vi "bbauv_acoustic_sbRIO_v3.vi"() -> ()   [LabVIEW 2012]
doc: "This VI will initialize the FPGA VI and read a user-defined number of samples from a DMA FIFO. When the data acquisition is complete this VI will read status information from the FPGA VI.\n\nFollow these instructions to run the VI.\n\n1. Select your RIO device from the dropdown.\n2. Set the sample period, number of samples to acquire per channel, and DMA block read size. \n\nNote: the block read size should be set to balance load on the host processor and the update rate of the user interface. A small block read size will update the user interface more often but will result in a higher load on the host processor."
uses:
  <vilib>/userdefined/High Color/nirio_resource_hc.ctl
  <vilib>/Analysis/3filter.llb/Filter Passband Type.ctl
  <vilib>/FPGAPlugInAG/sbRIO-9612/niLvFpga_Open_sbRIO-9612.vi
  <vilib>/rvi/interface/common/dynamic/niFpgaDynamicAddResources.vi
  <vilib>/Utility/error.llb/Error Cluster From Error Code.vi
  <vilib>/FPGAPlugInAG/Dynamic/niLvFpga_Run_Dynamic.vi
  <vilib>/rvi/errors/niLvFpgaAdjustHostInterfaceError.vi
  <vilib>/RVI Host/nirviSupport.llb/nirviErrorClusterFromErrorCode.vi
  <vilib>/FPGAPlugInAG/Dynamic/niLvFpga_Close_Dynamic.vi
  <vilib>/Analysis/3filter.llb/Elliptic Filter (DBL).vi
  <vilib>/Analysis/3filter.llb/Butterworth Filter (DBL).vi
  <vilib>/rvi/interface/nirviOpenFPGA/nirviOpenFPGA.xnode
  FPGA Bitfiles/bbauvFPGA_FPGATarget2_NI9223User-Contr_AXBjtBmtN8Y.lvbitx
  NI 9223 User-Controlled IO Sampling (FPGA).vi
  <vilib>/rvi/interface/nirviMethod/nirviMethod.xnode
  <vilib>/rvi/interface/nirviReadWriteControl/nirviReadWriteControl.xnode
  <vilib>/rvi/interface/nirviCloseFPGA/nirviCloseFPGA.xnode
  <vilib>/rvi/errors/niLvFpgaMergeErrorWithErrorCode.vi
  <vilib>/rvi/interface/Simulation/niFpgaSimulationCallBeginRW.vi
  <vilib>/FPGAPlugInAG/Dynamic/niLvFpga_ReadFifo_Dynamic.vi
  <vilib>/rvi/interface/nirviMethod/StockFPGA_InlinedMethodWaitForSingleIRQ.vi
  <vilib>/FPGAPlugInAG/Dynamic/niLvFpga_WaitOnIrq_Dynamic.vi
  <vilib>/FPGAPlugInAG/Dynamic/niLvFpga_AcknowledgeIrq_Dynamic.vi
  NiFpgaLv.dll
  <vilib>/FPGAPlugInAG/Dynamic/niLvFpga_ConfigureFifo_Dynamic.vi
  <vilib>/FPGAPlugInAG/Dynamic/niLvFpga_StartFifo_Dynamic.vi
  <vilib>/Analysis/NI_AALBase.lvlib
panel:
  in  "Freq Lower Limit:":dbl=25000.0
  out "Selected Frequency:":dbl
  in  "Filter mode":enum16{"Elliptic", "Butterworth"}(ring)=enum."Butterworth"
  in  "Order":i32=3
  in  "Low Cutoff":dbl=20000.0
  in  "High Cutoff":dbl=26000.0
  in  "Freq Upper Limit:":dbl=25000.0
  out "Freq 2":dbl
  out "Freq 1":dbl
  in  "Noise length":i32=300
  out "Index 0":dbl
  out "Index 1":dbl
  out "Index 2":dbl
  out "Index 3":dbl
  out "amplitude 0":dbl
  out "amplitude 1":dbl
  out "amplitude 2":dbl
  out "amplitude 3":dbl
  in  "Portion Duration":i32=1000
  out "Threshold 0":dbl
  out "Threshold 1":dbl
  out "Threshold 2":dbl
  out "Threshold 3":dbl
  in  "threshold ratio":dbl=3.0
  in  "Display":bool
  in  "Sampling Duration (us)":u32=2005000
  in  "RIO Device":T1="RIO0"
  out "Timed Out":bool
  out "Sample Gated":bool
  out "Overwrite":bool
  in  "Acquisition Stop":bool
  out "Selected Index":i32
  out "Ratio at Index (%)":dbl
  in  "Threshold":dbl=0.3
  out "Original Filtered Ch0":dbl[](graph)
  out "bad signal?":bool
  out "dt1":dbl
  out "dt2":dbl
  out "dt3":dbl
  out "ROS  Error":bool
  in  "Send to ROS":bool=TRUE
  in  "Altitude":dbl=2.0
  out "x":dbl
  out "y":dbl
  out "z":dbl
  out "yaw":dbl
  out "pitch":dbl
  in  "Mode":T2(ring)=enum."Use Far Field"
  out "Forward":dbl
  out "Sidemove":dbl
  out "Arrival Analysis Signal":dbl[][](graph)
  out "Yaw Chart":dbl(graph)
  out "noise index":dbl[](array[numeric])
  out "Frequency Selected Signal":dbl[](graph)
  out "#Elements Acquired":u32(graph)
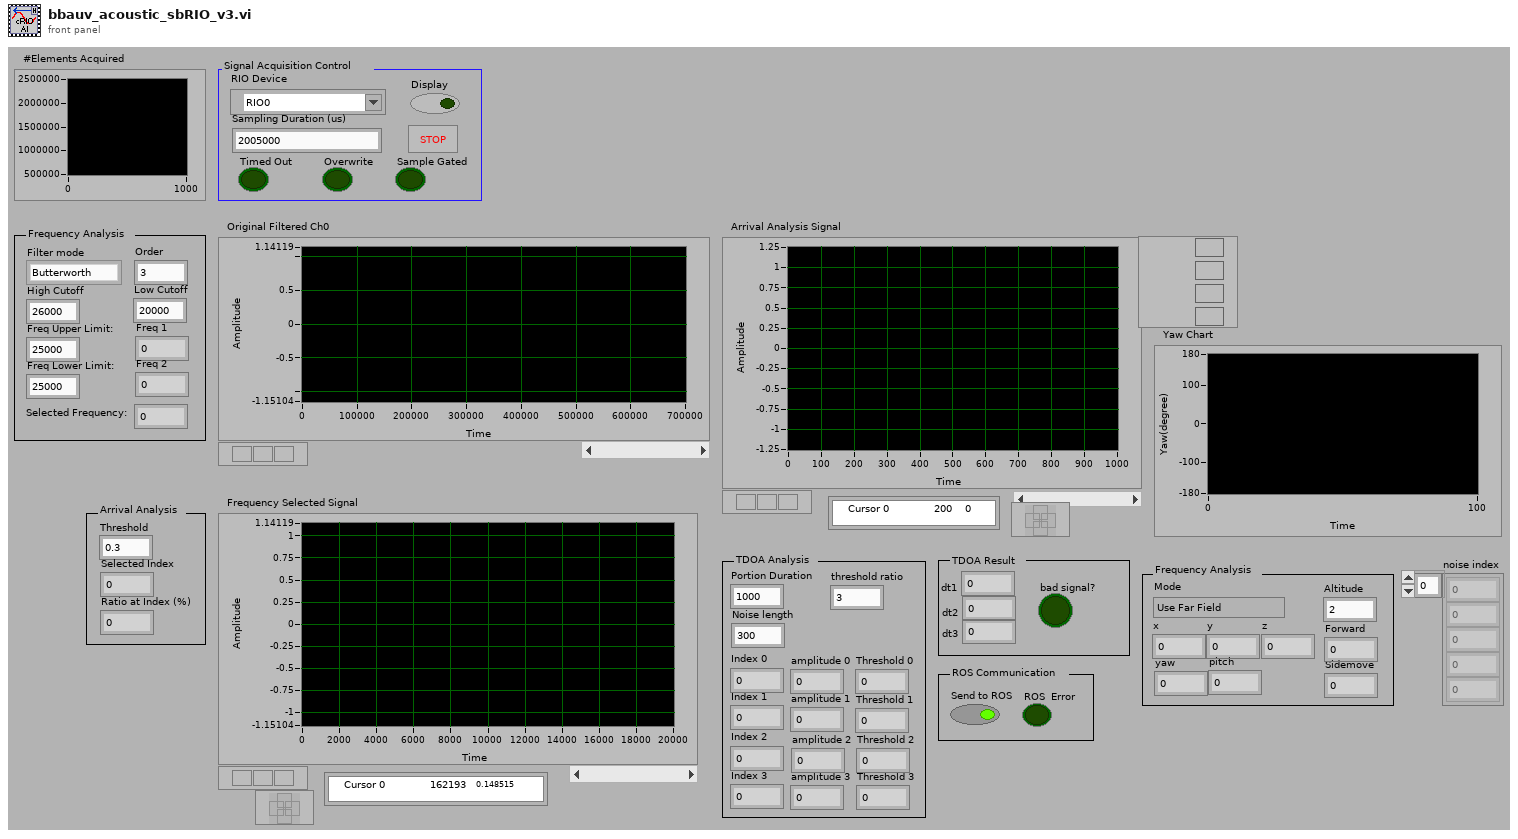
[diagram p1: front panel]
types:
  T1 = typedef "nirio_resource_hc.ctl" = tag
  T2 = enum16{"Use Near Field", "Use Far Field", "Far Field with 3 hydrophones"}
  T3 = typedef "NI_AALBase.lvlib/Filter Passband Type.ctl" = enum32{"Lowpass", "Highpass", "Bandpass", "Bandstop"}
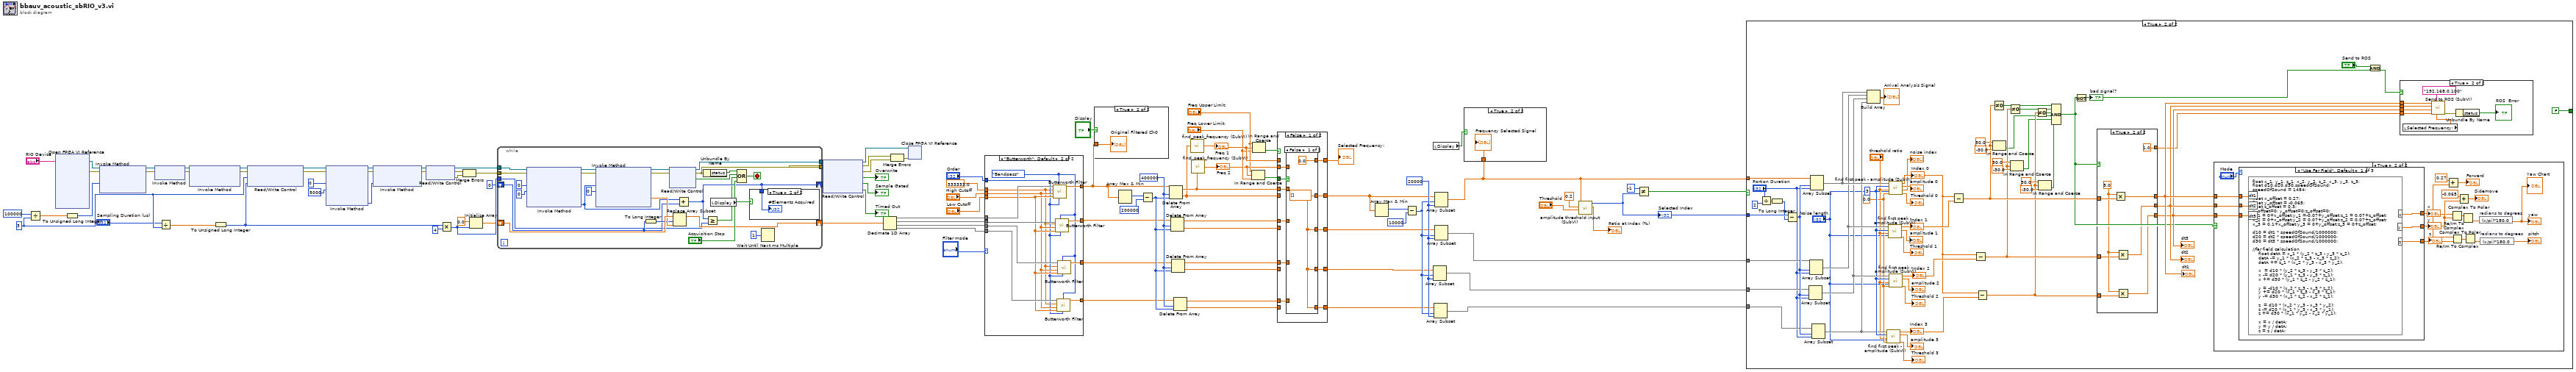
[diagram p0: block diagram]
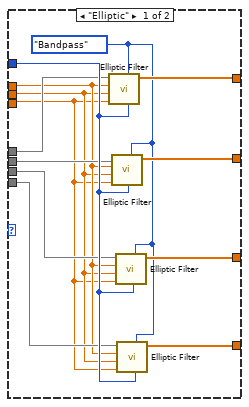
[diagram p6: hidden frame]
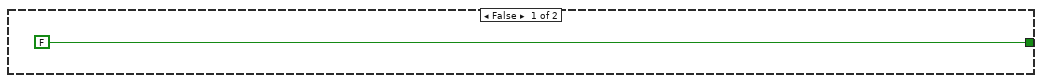
[diagram p7: hidden frame]
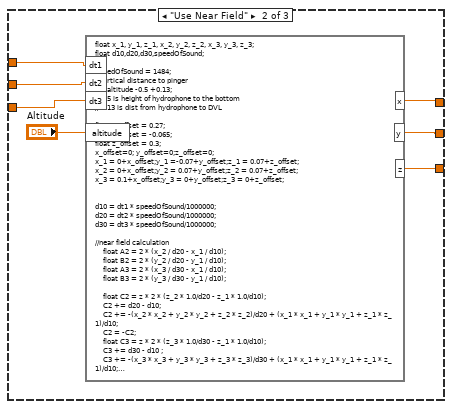
[diagram p9: hidden frame]
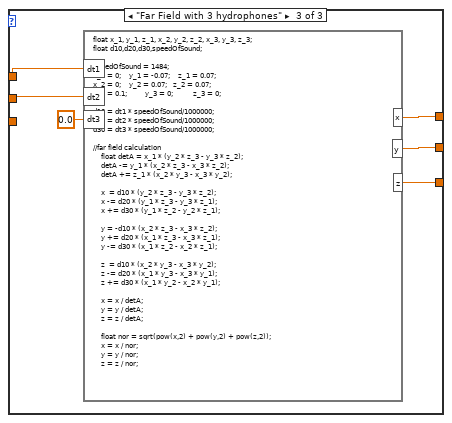
[diagram p10: hidden frame]
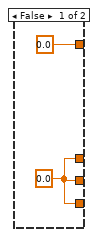
[diagram p12: hidden frame]
diagram:
  w46 = 20000
  w50 = 400000
  w57 = u32 3
  n1 = Divide(x=u32 100000, y=w57) -> (x/y=w90:dbl)
  n2 = xnode "Open FPGA VI Reference"("resource name"="RIO Device") -> ("FPGA VI Reference Out"=w93:refnum<k20>, "error out"=w92:errorcluster)  [unwired: 1 in]
  n3 = To Unsigned Long Integer(number=w90) -> (unsigned 32bit integer=w91:u32)
  n4 = xnode "Invoke Method"("FPGA VI Reference In"=w93, "error in"=w92, "Requested Depth"=w91) -> ("FPGA VI Reference Out"=w95:refnum<k20>, "error out"=w94:errorcluster)  [unwired: 1 out]
  n5 = xnode "Invoke Method"("FPGA VI Reference In"=w95, "error in"=w94) -> ("FPGA VI Reference Out"=w84:refnum<k20>, "error out"=w83:errorcluster)
  n6 = Divide(x="Sampling Duration (us)", y=w57) -> (x/y=w55:dbl)
  n7 = xnode "Invoke Method"("FPGA VI Reference In"=w84, "error in"=w83) -> ("FPGA VI Reference Out"=w60:refnum<k20>, "error out"=w59:errorcluster)  [unwired: 1 in]
  n8 = To Unsigned Long Integer(number=w55) -> (unsigned 32bit integer=w53:u32)
  n9 = xnode "Read/Write Control"("FPGA VI Reference In"=w60, "error in"=w59, "Sample Period (uSec)"=w57, "Number of Samples"=w53) -> ("FPGA VI Reference Out"=w74:refnum<k20>, "error out"=w73:errorcluster)
  n10 = xnode "Invoke Method"("FPGA VI Reference In"=w74, "error in"=w73, "IRQ Number(s)"=0, "Timeout (ms)"=5000) -> ("FPGA VI Reference Out"=w71:refnum<k20>, "error out"=w72:errorcluster, "IRQ(s) Asserted"=w68:i32)  [unwired: 1 out]
  n11 = xnode "Invoke Method"("FPGA VI Reference In"=w71, "error in"=w72, "IRQ Number(s)"=w68) -> ("FPGA VI Reference Out"=w70:refnum<k20>, "error out"=w69:errorcluster)
  n12 = xnode "Read/Write Control"("FPGA VI Reference In"=w70, "error in"=w69) -> ("FPGA VI Reference Out"=w62:refnum<k20>, "error out"=w76:errorcluster, "Error Out"=w75:errorcluster)
  n13 = Multiply(x=w53, y=u32 4) -> (x*y=w87:u32)
  n14 = Merge Errors(w76, w75) -> (w61:errorcluster)
  n15 = Initialize Array(sgl 0.0, w87) -> (w63:sgl[])
  n16 = while {
    tunnel: w62 -> [w109]
    tunnel: w61 -> [w108]
    tunnel: [w117] -> w82
    tunnel: [w116] -> w81
    shift-right: [w99] -> _
    shift-left: u32 0 -> [w110]
    tunnel: w87 -> [w102]
    shift-right: [w112] -> w54
    shift-left: w63 -> [w118]
    stop <- w119 stop-if-true
    n17 = xnode "Invoke Method"("FPGA VI Reference In"=w109, "error in"=w108, "Number of Elements"=u32 0, "Timeout (ms)"=0) -> ("FPGA VI Reference Out"=w107:refnum<k20>, "error out"=w106:errorcluster, "Elements Remaining"=w100:u32)  [unwired: 1 out]
    n18 = xnode "Invoke Method"("FPGA VI Reference In"=w107, "error in"=w106, "Number of Elements"=w100, "Timeout (ms)"=0) -> ("FPGA VI Reference Out"=w122:refnum<k20>, "error out"=w121:errorcluster, "Data"=w113:sgl[])  [unwired: 1 out]
    n19 = To Long Integer(number=w110) -> (32bit integer=w111:i32)
    n20 = xnode "Read/Write Control"("FPGA VI Reference In"=w122, "error in"=w121) -> ("FPGA VI Reference Out"=w117:refnum<k20>, "error out"=w116:errorcluster, "Error"=w101:bool)  [unwired: 1 out]
    n21 = Replace Array Subset(array=w118, new element=w113, index=w111) -> (w112:sgl[])
    n22 = Add(x=w100, y=w110) -> (x+y=w99:u32)
    n23 = Unbundle By Name(w116) -> ("status"=w103:bool)
    n24 = Greater Or Equal?(x=w99, y=w102) -> (x >= y?=w98:bool)
    n25 = local read "Display"() -> (w97:bool)
    n26 = Compound Arithmetic op=OR(w103, w101, w98, "Acquisition Stop") -> (w119:bool)
    n27 = case shown="True" w97 {
      tunnel: w99 -> [_ w123]
      frame False {
      }
      frame True {
        "#Elements Acquired" <- w123
      }
    }
    n28 = Wait Until Next ms Multiple(millisecond multiple=u32 1) -> ()  [unwired: 1 out]
  }
  n29 = xnode "Read/Write Control"("FPGA VI Reference In"=w82, "error in"=w81) -> ("FPGA VI Reference Out"=w86:refnum<k20>, "error out"=w77:errorcluster, "Error Out"=w78:errorcluster, "Overwrite"=→"Overwrite":bool, "Sample Gated"=→"Sample Gated":bool, "Timed Out"=→"Timed Out":bool)
  n30 = Decimate 1D Array(w54) -> (w22:sgl[], w32:sgl[], w33:sgl[], w31:sgl[])
  n31 = Merge Errors(w77, w78) -> (w85:errorcluster)
  n32 = xnode "Close FPGA VI Reference"("FPGA VI Reference In"=w86, "error in"=w85) -> ()  [unwired: 1 out]
  n33 = case shown="\"Butterworth\", Default" "Filter mode" {
    tunnel: w32 -> [w130 w149]
    tunnel: w31 -> [w128 w148]
    tunnel: w33 -> [w129 w147]
    tunnel: w22 -> [w131 w146]
    tunnel: [w136 w145] -> w23
    tunnel: [w135 w144] -> w26
    tunnel: [w134 w143] -> w25
    tunnel: [w133 w142] -> w24
    tunnel: "Low Cutoff" -> [w124 w141]
    tunnel: "High Cutoff" -> [w125 w140]
    tunnel: "Order" -> [w132 w139]
    tunnel: 333333.0 -> [w126 w138]
    frame "Elliptic" {
      w127 = Filter_Passband_Type."Bandpass"
      n34 = call-poly <vilib>:"Elliptic Filter.vi"("order"=w132, "filter type"=w127, "low cutoff freq: fl"=w124, "high cutoff freq: fh"=w125, "sampling freq: fs"=w126, "X"=w131) -> ("Filtered X"=w136:dbl[])  [unwired: 4 in, 1 out]
      n35 = call-poly <vilib>:"Elliptic Filter.vi"("order"=w132, "filter type"=w127, "low cutoff freq: fl"=w124, "high cutoff freq: fh"=w125, "sampling freq: fs"=w126, "X"=w130) -> ("Filtered X"=w135:dbl[])  [unwired: 4 in, 1 out]
      n36 = call-poly <vilib>:"Elliptic Filter.vi"("order"=w132, "filter type"=w127, "low cutoff freq: fl"=w124, "high cutoff freq: fh"=w125, "sampling freq: fs"=w126, "X"=w129) -> ("Filtered X"=w134:dbl[])  [unwired: 4 in, 1 out]
      n37 = call-poly <vilib>:"Elliptic Filter.vi"("order"=w132, "filter type"=w127, "low cutoff freq: fl"=w124, "high cutoff freq: fh"=w125, "sampling freq: fs"=w126, "X"=w128) -> ("Filtered X"=w133:dbl[])  [unwired: 4 in, 1 out]
    }
    frame "Butterworth", Default {
      w137 = Filter_Passband_Type."Bandpass"
      n38 = call-poly <vilib>:"Butterworth Filter.vi"("order"=w139, "filter type"=w137, "low cutoff freq: fl"=w141, "high cutoff freq: fh"=w140, "sampling freq: fs"=w138, "X"=w146) -> ("Filtered X"=w145:dbl[])  [unwired: 2 in, 1 out]
      n39 = call-poly <vilib>:"Butterworth Filter.vi"("order"=w139, "filter type"=w137, "low cutoff freq: fl"=w141, "high cutoff freq: fh"=w140, "sampling freq: fs"=w138, "X"=w149) -> ("Filtered X"=w144:dbl[])  [unwired: 2 in, 1 out]
      n40 = call-poly <vilib>:"Butterworth Filter.vi"("order"=w139, "filter type"=w137, "low cutoff freq: fl"=w141, "high cutoff freq: fh"=w140, "sampling freq: fs"=w138, "X"=w148) -> ("Filtered X"=w142:dbl[])  [unwired: 2 in, 1 out]
      n41 = call-poly <vilib>:"Butterworth Filter.vi"("order"=w139, "filter type"=w137, "low cutoff freq: fl"=w141, "high cutoff freq: fh"=w140, "sampling freq: fs"=w138, "X"=w147) -> ("Filtered X"=w143:dbl[])  [unwired: 2 in, 1 out]
    }
  }
  n42 = case shown="True" "Display" {
    tunnel: w23 -> [_ w150]
    frame False {
    }
    frame True {
      "Original Filtered Ch0" <- w150
    }
  }
  n43 = Array Max & Min(array=w23) -> (max index (indices)=w52:i32)  [unwired: 3 out]
  n44 = Subtract(x=w52, y=200000) -> (x-y=w49:i32)
  n45 = Delete From Array(array=w23, length=w50, index=w49) -> (deleted portion=w11:dbl[], array with subset deleted=w12:dbl[])
  n46 = Delete From Array(array=w26, length=w50, index=w49) -> (deleted portion=w9:dbl[], array with subset deleted=w10:dbl[])
  n47 = Delete From Array(array=w25, length=w50, index=w49) -> (deleted portion=w7:dbl[], array with subset deleted=w8:dbl[])
  n48 = Delete From Array(array=w24, length=w50, index=w49) -> (deleted portion=w5:dbl[], array with subset deleted=w6:dbl[])
  n49 = call "find_peak_frequency (SubVI).vi"("Signal"=w11) -> ("Frequency"=w13:dbl)
  "Freq 1" <- w13
  n50 = call "find_peak_frequency (SubVI).vi"("Signal"=w12) -> ("Frequency"=w1:dbl)
  "Freq 2" <- w1
  n51 = In Range and Coerce(upper limit="Freq Upper Limit:", x=w1, lower limit="Freq Lower Limit:") -> (In Range?=w19:bool)  [unwired: 1 out]
  n52 = In Range and Coerce(upper limit="Freq Upper Limit:", x=w13, lower limit="Freq Lower Limit:") -> (In Range?=w4:bool)  [unwired: 1 out]
  n53 = case shown="False" w4 {
    tunnel: w11 -> [_ w173]
    tunnel: w9 -> [_ w172]
    tunnel: w7 -> [_ w171]
    tunnel: w5 -> [_ w170]
    tunnel: w12 -> [w158 _]
    tunnel: w10 -> [w156 _]
    tunnel: w8 -> [w154 _]
    tunnel: w6 -> [w152 _]
    tunnel: [w157 w173] -> w17
    tunnel: [w155 w172] -> w16
    tunnel: [w153 w171] -> w15
    tunnel: [w151 w170] -> w14
    tunnel: [w159 w169] -> w18
    tunnel: w13 -> [_ w169]
    tunnel: w1 -> [w160 _]
    tunnel: w19 -> [w161 _]
    frame False {
      n54 = case shown="False" w161 {
        tunnel: w160 -> [_ w168]
        tunnel: [0.0 w168] -> w159
        tunnel: w158 -> [_ w167]
        tunnel: [w162 w167] -> w157
        tunnel: w156 -> [_ w166]
        tunnel: [w162 w166] -> w155
        tunnel: w154 -> [_ w165]
        tunnel: [w162 w165] -> w153
        tunnel: w152 -> [_ w164]
        tunnel: [w162 w164] -> w151
        frame False {
          w162 = dbl[] []
        }
        frame True {
        }
      }
    }
    frame True {
    }
  }
  "Selected Frequency:" <- w18
  n55 = Array Max & Min(array=w17) -> (max index (indices)=w47:i32)  [unwired: 3 out]
  n56 = Subtract(x=w47, y=10000) -> (x-y=w45:i32)
  n57 = local read "Display"() -> (w20:bool)
  n58 = Array Subset(array=w15, index=w45, length=w46) -> (w42:dbl[])
  n59 = Array Subset(array=w14, index=w45, length=w46) -> (w41:dbl[])
  n60 = Array Subset(array=w17, index=w45, length=w46) -> (w38:dbl[])
  n61 = Array Subset(array=w16, index=w45, length=w46) -> (w43:dbl[])
  n62 = case shown="True" w20 {
    tunnel: w38 -> [_ w174]
    frame False {
    }
    frame True {
      "Frequency Selected Signal" <- w174
    }
  }
  n63 = call "amplitude threshold input (SubVI).vi"("threshold"="Threshold", "%max amplitude"=0.2, "Array"=w38) -> ("actual ratio (%)"=→"Ratio at Index (%)":dbl, "Index"=w35:i32)  [unwired: 7 in]
  "Selected Index" <- w35
  n64 = Not Equal?(x=-1, y=w35) -> (x != y?=w40:bool)
  n65 = case shown="True" w40 {
    tunnel: w43 -> [_ w230]
    tunnel: w42 -> [_ w229]
    tunnel: w41 -> [_ w228]
    tunnel: w38 -> [_ w227]
    tunnel: w35 -> [_ w226]
    tunnel: [FALSE FALSE] -> _
    frame False {
    }
    frame True {
      w195 = 0.0
      w200 = 3
      n66 = Divide(x="Portion Duration", y=2) -> (x/y=w223:dbl)
      n67 = To Long Integer(number=w223) -> (32bit integer=w222:i32)
      n68 = Subtract(x=w226, y=w222) -> (x-y=w231:i32)
      n69 = Array Subset(array=w229, index=w231, length="Portion Duration") -> (w201:dbl[])
      n70 = Array Subset(array=w230, index=w231, length="Portion Duration") -> (w205:dbl[])
      n71 = Array Subset(array=w227, index=w231, length="Portion Duration") -> (w207:dbl[])
      n72 = Array Subset(array=w228, index=w231, length="Portion Duration") -> (w199:dbl[])
      n73 = Build Array(w207, w205, w201, w199) -> (→"Arrival Analysis Signal":dbl[][])
      n74 = call "find first peak - amplitude (SubVI).vi"("Noise duration (units)"="Noise length", "Noise min (amplitude)"=w195, "threshold ratio"="threshold ratio", "peak width (units)"=w200, "Array"=w199) -> ("Peak threshold"=→"Threshold 3":dbl, "peak amplitude"=→"amplitude 3":dbl, "Index"=w198:dbl)  [unwired: 2 in, 2 out]
      "Index 3" <- w198
      n75 = call "find first peak - amplitude (SubVI).vi"("Noise duration (units)"="Noise length", "threshold ratio"="threshold ratio", "peak width (units)"=w200, "Array"=w205) -> ("Peak threshold"=→"Threshold 1":dbl, "peak amplitude"=→"amplitude 1":dbl, "Index"=w204:dbl)  [unwired: 3 in, 2 out]
      "Index 1" <- w204
      n76 = call "find first peak - amplitude (SubVI).vi"("Noise duration (units)"="Noise length", "Noise min (amplitude)"=w195, "threshold ratio"="threshold ratio", "peak width (units)"=w200, "Array"=w207) -> ("Peak threshold"=→"Threshold 0":dbl, "noise index"=→"noise index":dbl[], "peak amplitude"=→"amplitude 0":dbl, "Index"=w194:dbl)  [unwired: 2 in, 1 out]
      "Index 0" <- w194
      n77 = call "find first peak - amplitude (SubVI).vi"("Noise duration (units)"="Noise length", "Noise min (amplitude)"=w195, "threshold ratio"="threshold ratio", "peak width (units)"=w200, "Array"=w201) -> ("Peak threshold"=→"Threshold 2":dbl, "peak amplitude"=→"amplitude 2":dbl, "Index"=w202:dbl)  [unwired: 2 in, 2 out]
      "Index 2" <- w202
      n78 = Subtract(x=w194, y=w204) -> (x-y=w185:dbl)
      n79 = Subtract(x=w194, y=w202) -> (x-y=w184:dbl)
      n80 = Subtract(x=w194, y=w198) -> (x-y=w183:dbl)
      n81 = Not Equal To 0?(x=w185) -> (x != 0?=w182:bool)
      n82 = In Range and Coerce(upper limit=30.0, x=w185, lower limit=-30.0) -> (In Range?=w179:bool)  [unwired: 1 out]
      n83 = Not Equal To 0?(x=w184) -> (x != 0?=w181:bool)
      n84 = In Range and Coerce(upper limit=30.0, x=w184, lower limit=-30.0) -> (In Range?=w178:bool)  [unwired: 1 out]
      n85 = Not Equal To 0?(x=w183) -> (x != 0?=w180:bool)
      n86 = In Range and Coerce(upper limit=30.0, x=w183, lower limit=-30.0) -> (In Range?=w177:bool)  [unwired: 1 out]
      n87 = Compound Arithmetic op=AND(w182, w181, w180, w179, w178, w177) -> (w176:bool)
      n88 = Not(x=w176) -> (.not. x?=→"bad signal?":bool)
      n89 = case shown="True" w176 {
        tunnel: w185 -> [_ w285]
        tunnel: w184 -> [_ w283]
        tunnel: w183 -> [_ w282]
        tunnel: [w276 w281] -> w212
        tunnel: [w276 w280] -> w211
        tunnel: [w276 w279] -> w210
        tunnel: [0.0 1.0] -> w209
        frame False {
          w276 = 0.0
        }
        frame True {
          w284 = 3.0
          n90 = Multiply(x=w284, y=w285) -> (x*y=w281:dbl)
          n91 = Multiply(x=w284, y=w283) -> (x*y=w280:dbl)
          n92 = Multiply(x=w284, y=w282) -> (x*y=w279:dbl)
        }
      }
      "dt1" <- w212
      "dt2" <- w211
      "dt3" <- w210
      n93 = case shown="True" w176 {
        tunnel: w212 -> [_ w240]
        tunnel: w211 -> [_ w239]
        tunnel: w210 -> [_ w238]
        frame False {
        }
        frame True {
          n94 = case shown="\"Use Far Field\", Default" "Mode" {
            tunnel: [w254 w261 w266] -> w232
            tunnel: [w253 w260 w265] -> w235
            tunnel: [w252 w259 w264] -> w244
            tunnel: w240 -> [w251 w257 w263]
            tunnel: w239 -> [w250 w256 w262]
            tunnel: w238 -> [w249 w255 _]
            frame "Use Far Field", Default {
              n95 = formula code="float x_1, y_1, z_1, x_2, y_2, z_2, x_3, y_3, z_3;\nfloat d10,d20,d30,speedOfSound;\nspeedOfSound = 1484;\n\nfloat x_offset = 0.27;\nfloat y_offset = -0.065;\nfloat z_offset = 0.3;\nx_offset=0; y_offset=0;z_offset=0;\nx_1 = 0+x_offset;y_1 =-0.07+y_offset;z_1 = 0.07+z_offset;\nx_2 = 0+x_offset;y_2 = 0.07+y_offset;z_2 = 0.07+z_offset;\nx_3 = 0.1+x_offset;y_3 = 0+y_offset;z_3 = 0+z_offset;\n\nd10 = dt1 * speedOfSound/1000000;\nd20 = dt2 * speedOfSound/1000000;\nd30 = dt3 * speedOfSound/1000000;\n\n//far field calculation\n    float detA = x_1 * (y_2 * z_3 - y_3 * z_2);\n    detA -= y_1 * (x_2 * z_3 - x_3 * z_2);\n    detA += z_1 * (x_2 * y_3 - x_3 * y_2);\n\n    x  = d10 * (y_2 * z_3 - y_3 * z_2);\n    x -= d20 * (y_1 * z_3 - y_3 * z_1);\n    x += d30 * (y_1 * z_2 - y_2 * z_1);\n\n    y = -d10 * (x_2 * z_3 - x_3 * z_2);\n    y += d20 * (x_1 * z_3 - x_3 * z_1);\n    y -= d30 * (x_1 * z_2 - x_2 * z_1);\n\n    z  = d10 * (x_2 * y_3 - x_3 * y_2);\n    z -= d20 * (x_1 * y_3 - x_3 * y_1);\n    z += d30 * (x_1 * y_2 - x_2 * y_1);\n\n    x = x / detA;\n    y = y / detA;\n    z = z / detA;\n\n    float nor = sqrt(pow(x,2) + pow(y,2) + pow(z,2));\n    x = x / nor;\n    y = y / nor;\n    z = z / nor;"("dt1"=w251, "dt2"=w250, "dt3"=w249) -> ("x"=w254:dbl, "y"=w253:dbl, "z"=w252:dbl)
            }
            frame "Use Near Field" {
              n96 = formula code="float x_1, y_1, z_1, x_2, y_2, z_2, x_3, y_3, z_3;\nfloat d10,d20,d30,speedOfSound;\n\nspeedOfSound = 1484;\n//vertical distance to pinger\nz= altitude -0.5 +0.13;\n// 0.5 is height of hydrophone to the bottom\n// 0.13 is dist from hydrophone to DVL\n\nfloat x_offset = 0.27;\nfloat y_offset = -0.065;\nfloat z_offset = 0.3;\nx_offset=0; y_offset=0;z_offset=0;\nx_1 = 0+x_offset;y_1 =-0.07+y_offset;z_1 = 0.07+z_offset;\nx_2 = 0+x_offset;y_2 = 0.07+y_offset;z_2 = 0.07+z_offset;\nx_3 = 0.1+x_offset;y_3 = 0+y_offset;z_3 = 0+z_offset;\n\n\nd10 = dt1 * speedOfSound/1000000;\nd20 = dt2 * speedOfSound/1000000;\nd30 = dt3 * speedOfSound/1000000;\n\n//near field calculation\n    float A2 = 2 * (x_2 / d20 - x_1 / d10);\n    float B2 = 2 * (y_2 / d20 - y_1 / d10);\n    float A3 = 2 * (x_3 / d30 - x_1 / d10);\n    float B3 = 2 * (y_3 / d30 - y_1 / d10);\n    \n    float C2 = z * 2 * (z_2 * 1.0/d20 - z_1 * 1.0/d10);\n    C2 += d20 - d10;\n    C2 += -(x_2 * x_2 + y_2 * y_2 + z_2 * z_2)/d20 + (x_1 * x_1 + y_1 * y_1 + z_1 * z_1)/d10;\n    C2 = -C2;\n    float C3 = z * 2 * (z_3 * 1.0/d30 - z_1 * 1.0/d10);\n    C3 += d30 - d10 ;\n    C3 += -(x_3 * x_3 + y_3 * y_3 + z_3 * z_3)/d30 + (x_1 * x_1 + y_1 * y_1 + z_1 * z_1)/d10;\n    C3 = -C3;\n\n    if (A2*B3 == A3*B2) {\n        x = 0;\n        y = 0;\n    }\n    else {\n        x = (C2 * B3 - C3 * B2) / (A2 * B3 - A3 * B2);\n        y = (C3 * A2 - C2 * A3) / (B3 * A2 - B2 * A3);\n    }"("dt1"=w257, "dt2"=w256, "dt3"=w255, "altitude"="Altitude") -> ("x"=w261:dbl, "y"=w260:dbl, "z"=w259:dbl)
            }
            frame "Far Field with 3 hydrophones" {
              n97 = formula code="float x_1, y_1, z_1, x_2, y_2, z_2, x_3, y_3, z_3;\nfloat d10,d20,d30,speedOfSound;\n\nspeedOfSound = 1484;\nx_1 = 0;    y_1 = -0.07;    z_1 = 0.07;\nx_2 = 0;    y_2 = 0.07;   z_2 = 0.07;\nx_3 = 0.1;         y_3 = 0;          z_3 = 0;\n\nd10 = dt1 * speedOfSound/1000000;\nd20 = dt2 * speedOfSound/1000000;\nd30 = dt3 * speedOfSound/1000000;\n\n//far field calculation\n    float detA = x_1 * (y_2 * z_3 - y_3 * z_2);\n    detA -= y_1 * (x_2 * z_3 - x_3 * z_2);\n    detA += z_1 * (x_2 * y_3 - x_3 * y_2);\n\n    x  = d10 * (y_2 * z_3 - y_3 * z_2);\n    x -= d20 * (y_1 * z_3 - y_3 * z_1);\n    x += d30 * (y_1 * z_2 - y_2 * z_1);\n\n    y = -d10 * (x_2 * z_3 - x_3 * z_2);\n    y += d20 * (x_1 * z_3 - x_3 * z_1);\n    y -= d30 * (x_1 * z_2 - x_2 * z_1);\n\n    z  = d10 * (x_2 * y_3 - x_3 * y_2);\n    z -= d20 * (x_1 * y_3 - x_3 * y_1);\n    z += d30 * (x_1 * y_2 - x_2 * y_1);\n\n    x = x / detA;\n    y = y / detA;\n    z = z / detA;\n\n    float nor = sqrt(pow(x,2) + pow(y,2) + pow(z,2));\n    x = x / nor;\n    y = y / nor;\n    z = z / nor;"("dt1"=w263, "dt2"=w262, "dt3"=0.0) -> ("x"=w266:dbl, "y"=w265:dbl, "z"=w264:dbl)
            }
          }
          "x" <- w232
          "y" <- w235
          "z" <- w244
          n98 = Add(x=0.27, y=w232) -> (x+y=→"Forward":dbl)
          n99 = Re/Im To Complex(1:w235, 2:w232) -> (0:w242:cdb)
          n100 = Re/Im To Complex(1:w244, 2:w232) -> (0:w245:cdb)
          n101 = Add(x=-0.065, y=w235) -> (x+y=→"Sidemove":dbl)
          n102 = Complex To Polar(r * e^(i*theta)=w242) -> (theta=w243:dbl)  [unwired: 1 out]
          n103 = Complex To Polar(r * e^(i*theta)=w245) -> (theta=w247:dbl)  [unwired: 1 out]
          n104 = expression code="(x/pi)*180.0"(w243) -> (→"yaw" →"Yaw Chart":dbl)
          n105 = expression code="(x/pi)*180.0"(w247) -> (→"pitch":dbl)
        }
      }
      n106 = And(x="Send to ROS", y=w176) -> (x .and. y?=w208:bool)
      n107 = case shown="True" w208 {
        tunnel: w212 -> [_ w272]
        tunnel: w211 -> [_ w271]
        tunnel: w210 -> [_ w270]
        tunnel: w209 -> [_ w269]
        frame False {
        }
        frame True {
          n108 = local read "Selected Frequency:"() -> (w268:dbl)
          n109 = call "Send to ROS (SubVI).vi"("frequency"=w268, "ROS IP"="192.168.0.100", "Good signal?"=w269, "dt 3"=w270, "dt2"=w271, "dt 1"=w272) -> ("error out"=w274:errorcluster)  [unwired: 5 in]
          n110 = Unbundle By Name(w274) -> ("status"=→"ROS  Error":bool)
        }
      }
    }
  }
